vi "MoveBySteps.vi"(6 "Direction":enum16{"Forward", "Backwards"}(ring), 7 "Polarity":enum16{"Positive", "Negative"}(ring), 8 "error in (no error)":errorcluster, 9 "Speed":u32, 10 "Steps":enum32{""}(ring), 11 "TranslationStage in":refnum<class "ArduinoTranslationStage.lvclass">) -> (0 "error out":errorcluster, 3 "TranslationStage out":refnum<class "ArduinoTranslationStage.lvclass">)   [LabVIEW 2023, in "ArduinoTranslationStage.lvlib" / "ArduinoTranslationStage.lvclass"]
uses:
  ArduinoTranslationStage.lvclass
  ArduinoTranslationStage.lvclass/ArduinoTranslationStage.ctl
  <vilib>/Instr/_visa.llb/Select Event Type.ctl
  TranslationStagesComm Messages/StageMoveDone Msg/StageMoveDone Msg.lvclass
  <vilib>/ActorFramework/Actor/Actor.lvclass
  Applications/National Instruments/LabVIEW 2023 64-bit/vi.lib/ActorFramework/Actor/Actor.lvclass
  Users/alexandrosspiliotis/Documents/TranslationStage/ArduinoTranslationStageActor/ArduinoTranslationStage Actor/ArduinoTranslationStage.lvclass
  Users/alexandrosspiliotis/Documents/Cameras_LV/InitDeinit/InitDeinit.lvclass
  Users/alexandrosspiliotis/Documents/TranslationStage/StepperMotorController/StepperMotorController.lvclass
  Users/alexandrosspiliotis/Documents/TranslationStage/TranslationStages/TranslationStagesInterface.lvclass
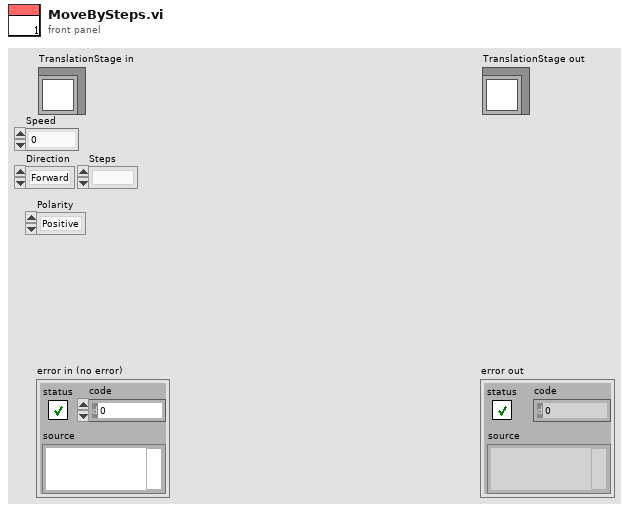
[diagram p1: front panel]
types:
  T1 = typedef "Select Event Type.ctl" = u32
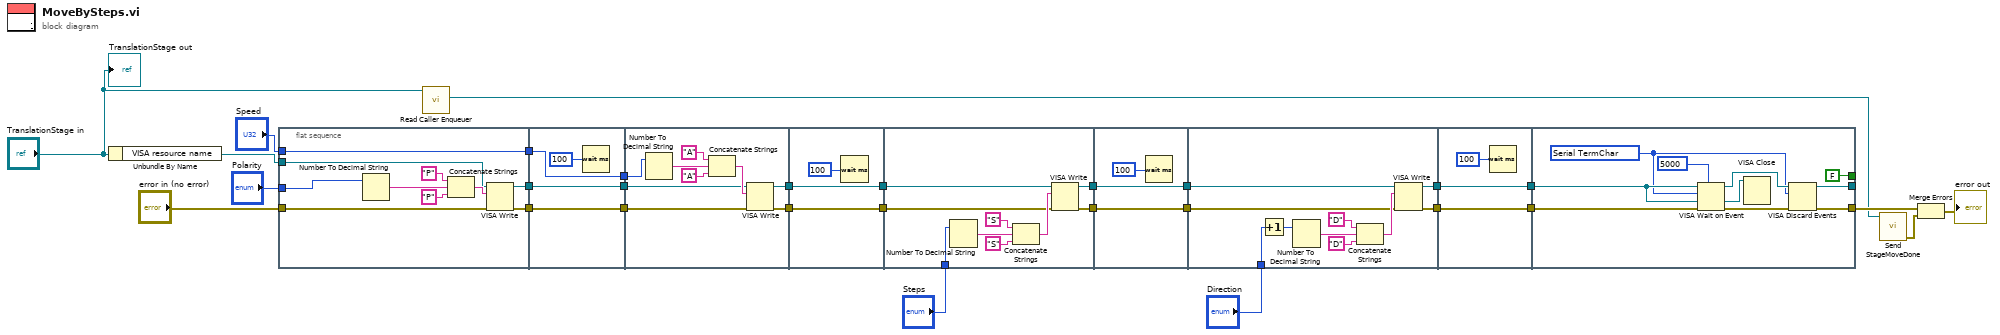
[diagram p0: block diagram]
diagram:
  n1 = Unbundle By Name("TranslationStage in") -> ("VISA resource name"=w6:refnum<visa-resource-name>)
  n2 = flat-sequence {
    tunnel: w6 -> [w31]
    tunnel: "Speed" -> [w39]
    tunnel: "error in (no error)" -> [w35]
    tunnel: [w34] -> w29
    tunnel: [w39] -> w28
    tunnel: [w32] -> w27
    tunnel: "Polarity" -> [w30]
    tunnel: [w43] -> w26
    tunnel: [w42] -> w25
    tunnel: [w41] -> w24
    tunnel: w29 -> [w43]
    tunnel: w28 -> [w42]
    tunnel: w27 -> [w41]
    tunnel: [w48] -> w23
    tunnel: [w44] -> w22
    tunnel: w26 -> [w50]
    tunnel: w25 -> [w46]
    tunnel: w24 -> [w45]
    tunnel: [w54] -> w21
    tunnel: w23 -> [w54]
    tunnel: [w53] -> w20
    tunnel: w22 -> [w53]
    tunnel: w21 -> [w61]
    tunnel: [w60] -> w18
    tunnel: [w58] -> w19
    tunnel: "Steps" -> [w57]
    tunnel: w20 -> [w56]
    tunnel: [w67] -> w17
    tunnel: [w66] -> w16
    tunnel: w19 -> [w66]
    tunnel: w18 -> [w67]
    tunnel: [w77] -> w15
    tunnel: [w76] -> w14
    tunnel: w17 -> [w69]
    tunnel: w16 -> [w70]
    tunnel: "Direction" -> [w68]
    tunnel: w15 -> [w80]
    tunnel: w14 -> [w79]
    tunnel: [w80] -> w12
    tunnel: [w79] -> w13
    tunnel: w13 -> [w87]
    tunnel: w12 -> [w90]
    tunnel: [w83] -> _
    tunnel: [w82] -> w5
    tunnel: [FALSE ("event data")] -> _
    frame #0 {
      n3 = Number To Decimal String(number=w30) -> (decimal integer string=w36:string)  [unwired: 1 in]
      n4 = Concatenate Strings("P" ("write buffer"), w36, "P" ("string")) -> (w37:string)
      n5 = VISA Write(VISA resource name=w31, write buffer=w37, error in (no error)=w35) -> (VISA resource name out=w32:refnum<visa-resource-name>, error out=w34:errorcluster)  [unwired: 1 out]
    }
    frame #1 {
      n6 = Wait (ms)(milliseconds to wait=u32 100) -> ()  [unwired: 1 out]
    }
    frame #2 {
      n7 = Number To Decimal String(number=w46) -> (decimal integer string=w47:string)  [unwired: 1 in]
      n8 = Concatenate Strings("A" ("write buffer"), w47, "A" ("string")) -> (w49:string)
      n9 = VISA Write(VISA resource name=w45, write buffer=w49, error in (no error)=w50) -> (VISA resource name out=w44:refnum<visa-resource-name>, error out=w48:errorcluster)  [unwired: 1 out]
    }
    frame #3 {
      n10 = Wait (ms)(milliseconds to wait=u32 100) -> ()  [unwired: 1 out]
    }
    frame #4 {
      n11 = Number To Decimal String(number=w57) -> (decimal integer string=w59:string)  [unwired: 1 in]
      n12 = Concatenate Strings("S" ("write buffer"), w59, "S" ("string")) -> (w62:string)
      n13 = VISA Write(VISA resource name=w56, write buffer=w62, error in (no error)=w61) -> (VISA resource name out=w58:refnum<visa-resource-name>, error out=w60:errorcluster)  [unwired: 1 out]
    }
    frame #5 {
      n14 = Wait (ms)(milliseconds to wait=u32 100) -> ()  [unwired: 1 out]
    }
    frame #6 {
      n15 = Increment(x=w68) -> (x+1=w72:enum16{"Forward", "Backwards"})
      n16 = Number To Decimal String(number=w72) -> (decimal integer string=w71:string)  [unwired: 1 in]
      n17 = Concatenate Strings("D" ("write buffer"), w71, "D" ("string")) -> (w74:string)
      n18 = VISA Write(VISA resource name=w70, write buffer=w74, error in (no error)=w69) -> (VISA resource name out=w76:refnum<visa-resource-name>, error out=w77:errorcluster)  [unwired: 1 out]
    }
    frame #7 {
      n19 = Wait (ms)(milliseconds to wait=u32 100) -> ()  [unwired: 1 out]
    }
    frame #8 {
      w84 = T1 1073684516 items=["Service Request"=1073684491, "Trigger"=3221168138, "Clear"=1073684493, "VXI Signal"=1073684512, "VXI/VME Interrupt"=3221168161, "VXI/VME Sysfail"=1073684509, "VXI/VME Sysreset"=1073684510, "GPIB CIC"=1073684498, "GPIB Talk"=1073684499, "GPIB Listen"=1073684500, "PXI Interrupt"=1073684514, "Serial Break"=1073684515, "Serial TermChar"=1073684516, "Serial CTS"=1073684521, "Serial DSR"=1073684522, "Serial DCD"=1073684524, "Serial RI"=1073684526, "Serial Character"=1073684533, "USB Interrupt"=1073684535, "All Enabled"=1073709055] ("Event Type")
      n20 = VISA Wait on Event(7:u32 5000 ("timeout (0)"), 8:w90, 9:w87, 10:w84, 11:w87) -> (0:w85:errorcluster, 1:w88:refnum<visa-resource-name>, 3:w86:refnum<visa-resource-name>)  [unwired: 1 out]
      n21 = VISA Close(VISA resource name=w88) -> ()  [unwired: 1 in, 1 out]
      n22 = VISA Discard Events(8:w85, 10:w84, 11:w86) -> (0:w82:errorcluster, 3:w83:refnum<visa-resource-name>)  [unwired: 1 in]
    }
  }
  n23 = call <vilib>:"Read Caller Enqueuer.vi"("Actor"="TranslationStage in") -> ("Caller Enqueuer"=w3:refnum<class "Message Enqueuer.lvclass">)  [unwired: 10 in]
  n24 = call "Send StageMoveDone.vi"("Message Enqueuer"=w3) -> ("error out"=w1:errorcluster)  [unwired: 9 in, 1 out]
  n25 = Merge Errors(w5, w1) -> (→"error out":errorcluster)
  "TranslationStage out" <- "TranslationStage in"
